vi "Get Pinmap Client.vi"(8 "error in (no error)":errorcluster, 11 "ClientPool in":refnum<class "gRPC Client Pool.lvclass">) -> (0 "error out":errorcluster, 2 "Pinmap grpc id":T1, 3 "ClientPool out":refnum<class "gRPC Client Pool.lvclass">)   [LabVIEW 2020, in "MeasurementLink gRPC Utilities.lvlib" / "gRPC Client Pool.lvclass"]
uses:
  gRPC Client Pool.lvclass
  <vilib>/gRPC/LabVIEW gRPC Library/Shared/grpcId.ctl
  gRPC Client Pool.lvclass/gRPC Client Pool.ctl
  MeasurementLink Discovery Client/RPC Messages/ni_measurementlink_discovery_v1_ResolveServiceRequest.ctl
  MeasurementLink Discovery Client/MeasurementLink Discovery Client.lvlib
  MeasurementLink Pin Map Client/MeasurementLink Pin Map Client.lvlib
  MeasurementLink gRPC Utilities.lvlib
  <vilib>/gRPC/LabVIEW gRPC Library/grpc-lvsupport-release.lvlib
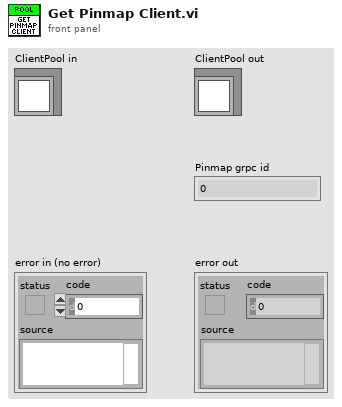
[diagram p1: front panel]
types:
  T1 = typedef "grpc-lvsupport-release.lvlib/grpcId.ctl" = u64
  T2 = typedef "MeasurementLink Discovery Client.lvlib/ni_measurementlink_discovery_v1_ResolveServiceRequest.ctl" = cluster{"provided_interface":string, "service_class":string}
  T3 = typedef "MeasurementLink Discovery Client.lvlib/ni_measurementlink_discovery_v1_ServiceLocation.ctl" = cluster{"location":string, "insecure_port":string, "ssl_authenticated_port":string}
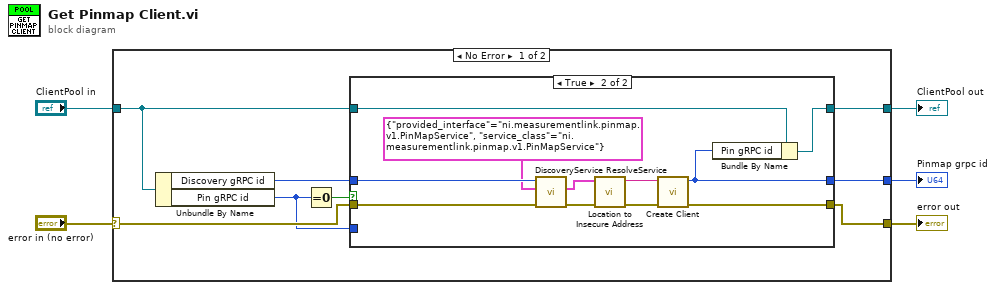
[diagram p0: block diagram]
diagram:
  n1 = case shown="No Error" "error in (no error)" {
    selector: "error in (no error)" -> [w11 w28]
    tunnel: [w10 w28] -> w4
    tunnel: [w8 w27] -> w2
    tunnel: "ClientPool in" -> [w6 w27]
    tunnel: [w9 _] -> w1
    frame No Error {
      n2 = Unbundle By Name(w6) -> ("Discovery gRPC id"=w12:T1, "Pin gRPC id"=w7:T1)
      n3 = Equal To 0?(x=w7) -> (x = 0?=w13:bool)
      n4 = case shown="True" w13 {
        tunnel: w12 -> [_ w25]
        tunnel: w11 -> [w16 w24]
        tunnel: [w15 w23] -> w9
        tunnel: [w16 w22] -> w10
        tunnel: w7 -> [w15 _]
        tunnel: w6 -> [w14 w18]
        tunnel: [w14 w17] -> w8
        frame False {
        }
        frame True {
          n5 = call "DiscoveryService ResolveService.vi"("error in"=w24, "Request Data"=T2 {"provided_interface"="ni.measurementlink.pinmap.v1.PinMapService", "service_class"="ni.measurementlink.pinmap.v1.PinMapService"}, "gRPC ID"=w25) -> ("error out"=w26:errorcluster, "Response Data"=w20:T3)  [unwired: 6 in, 1 out]
          n6 = call "Location to Insecure Address.vi"("Location"=w20) -> ("Address"=w19:string)  [unwired: 10 in]
          n7 = call "Create Client.vi"("error in"=w26, "address"=w19) -> ("error out"=w22:errorcluster, "gRPC ID Out"=w23:T1)  [unwired: 8 in]
          n8 = Bundle By Name(cluster=w18, "Pin gRPC id"=w23) -> (w17:refnum<class "gRPC Client Pool.lvclass">)
        }
      }
    }
    frame Error {
    }
  }
  "error out" <- w4
  "ClientPool out" <- w2
  "Pinmap grpc id" <- w1
